vi "F5xxx Close.vi"(8 "error in (no error)":errorcluster, 11 "session in":T1) -> (0 "error out":errorcluster, 3 "session out":T1)   [LabVIEW 2020]
doc: "Close Fluke 5xxx."
uses:
  F5xxx_session.ctl
  F5xxx_output_mode.ctl
  Fluke 5XXX Series Multicalibrators.lvlib
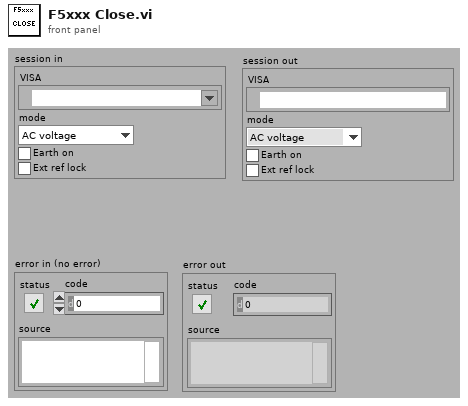
[diagram p1: front panel]
types:
  T1 = typedef "F5xxx_session.ctl" = cluster{"VISA":refnum<visa-resource-name>, "mode":T2, "Earth on":bool, "Ext ref lock":bool}
  T2 = typedef "F5xxx_output_mode.ctl" = enum16{"AC voltage", "AC current"}
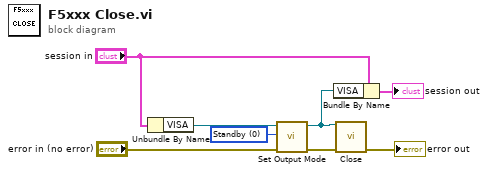
[diagram p0: block diagram]
diagram:
  w1 = u32 0 items=["Standby", "Operate"] ("Output Mode (0: Standby)")
  n1 = Unbundle By Name("session in") -> ("VISA"=w4:refnum<visa-resource-name>)
  n2 = call "Set Output Mode.vi"("error in (no error)"="error in (no error)", "Output Mode (0: Standby)"=w1, "VISA resource name"=w4) -> ("error out"=w5:errorcluster, "VISA resource name out"=w2:refnum<visa-resource-name>)  [unwired: 7 in]
  n3 = Bundle By Name(cluster="session in", "VISA"=w2) -> (→"session out":T1)
  n4 = call "Close.vi"("VISA resource name"=w2, "error in (no error)"=w5) -> ("error out"=→"error out":errorcluster)  [unwired: 13 in]
